vi "PCS Correlation_AVG.vi"() -> ()   [LabVIEW 2022 SP3]
uses:
  <vilib>/Analysis/baseanly.llb/Mean (DBL).vi
  <vilib>/Utility/file.llb/Write To Spreadsheet File (DBL).vi
  <vilib>/Utility/file.llb/Read From Spreadsheet File (DBL).vi
  <vilib>/Analysis/NI_AALBase.lvlib
panel:
  in  "Calc Angle":dbl=90.0
  in  "No motor":bool
  in  "No SPC":bool
  in  "stop":bool
  in  "Tab Control":T1(tab)
  out "G2 Exp Fit":cluster{dbl[], "Best Exponential Fit":dbl[]}[](graph)
  in  "AC length":i32=256
  in  "New File":bool
  in  "Total Time (s)":i32=100
  out "Time step (ms)":dbl
  in  "zero lag +":i32=1
  in  "Sample Rate (Hz)":dbl=100000.0
  in  "Data Source":enum16{"NI Card Grab", "NI File"}(ring)
  out "Cumulant ln fit":cluster{dbl[], "ln(x)/2":dbl[]}[](graph)
  out "Cumulant Fit":T2
  in  "Tau":u8
  out "bin mean":dbl format="%0.2f"
  out "Fit":T3
  out "SVM Size (um)":cluster{i32, "x":i32, dbl[][]}(graph)
  out "SVM Gaps":cluster{i32, "x":i32, dbl[][]}(graph)
  out "MultiTau":cluster{"Data out":dbl[], dbl[]}(graph)
  out "File Path":path
  out "SVM Fit Columns":T4(array[cluster])
  out "Means":dbl[](graph)
  out "Bin SD":dbl format="%0.2f"
  in  "Angle Index":u32
  out "Capture Angle":dbl
  in  "Save Path Root":path=path "D:/File"
  in  "SVs":u8
  in  "Save Bin Data":bool
  out "G2":dbl[][](graph)
  in  "Clear State":bool
  in  "angle plot":bool
  in  "Clear Chart":bool
  out "Polar Plot":picture
  out "Angle Plot":cluster{dbl[], dbl[]}(graph)
  in  "PC":T5={"Number of Bins"=1, "Bin Time (s)"=0.1, "Pause Time (s)"=1e-06}
  out "Bin Count":u32(graph)
  out "Counter":u32 caption="Counts/bin"
  out "APD saturation":bool
  in  "Run Angle collection":bool
  in  "Start":i16=90
  in  "# Steps":i16
  in  "Step Interval (degrees)":dbl=0.5 min=0.5 max=180.0 step=0.5
  out "Stop Angle":i32
  out "Current Step":i32
  out "cluster":T6
  in  "MG17Motor":refnum<k7>(container)
  in  "Diameter (um)":dbl=0.04
  out "Theory":T7
  in  "save mie":bool
  in  "Mie Input":T8={"wavlength (um)"=0.633, "Diameter (um)"=0.1, "n"=1.53, "pts"=1000.0, "Collection Angle"=4.0}
  out "Mie Theory (Matlab)":cluster{"angle":dbl[], "I":dbl[]}[](graph)
  # "SVM Method"
  # "Simple Decay Fit"
  # "Cumulant Method"
  # "Expected decay"
  # "`"
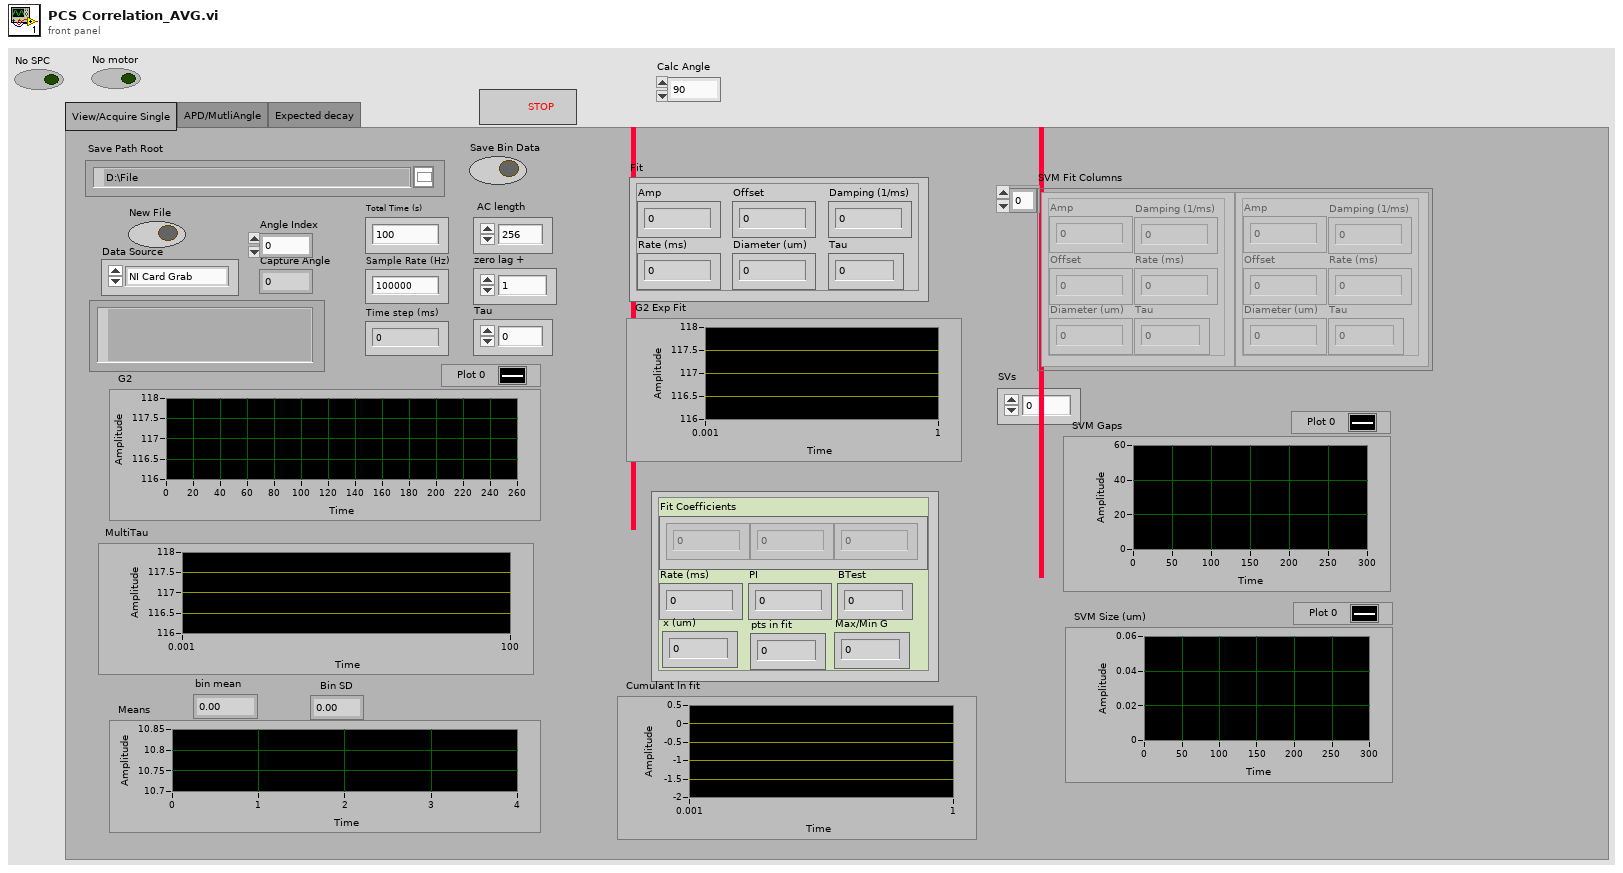
[diagram p1: front panel]
types:
  T1 = enum32{"View/Acquire Single", "APD/MutliAngle", "Expected decay"}
  T2 = cluster{"Fit Coefficients":dbl[], "Rate (ms)":dbl, "PI":dbl, "BTest":dbl, "x (um)":dbl, "pts in fit":dbl, "Max/Min G":dbl}
  T3 = cluster{"Amp":dbl, "Offset":dbl, "Damping (1/ms)":dbl, "Rate (ms)":dbl, "Diameter (um)":dbl, "Tau":dbl}
  T4 = cluster{"Amp":dbl, "Offset":dbl, "Damping (1/ms)":dbl, "Rate (ms)":dbl, "Diameter (um)":dbl, "Tau":dbl}[]
  T5 = cluster{"Number of Bins":i16, "Bin Time (s)":dbl, "Pause Time (s)":dbl}
  T6 = cluster{"running":bool, "gate active":bool, "waiting for trig":bool, "overflow":bool, "overload":bool, "overtemp":bool, "APD Sat b0":bool, "APD Sat bit1":bool, "N/A":bool, "N/A":bool, "overlow accum":bool, "overload accum":bool, "overtemp accum":bool, "APD Sat Accum 0":bool, "APD Sat Accum 0":bool}
  T7 = cluster{"Damping (1/ms)":dbl, "Rate (ms)":dbl, "Tau":dbl}
  T8 = cluster{"wavlength (um)":dbl, "Diameter (um)":dbl, "n":dbl, "pts":dbl, "Collection Angle":dbl}
  T9 = cluster{"G2 Array":dbl[][], "Sample Rate":dbl, "means":dbl[], "AC length":i32, "Total Time (s)":i32, "Angle":dbl}
  T10 = cluster{"maximum":dbl, "minimum":dbl, "clip to min":bool, "log?(F)":bool, "grid color":u32, "plot color":u32, "fmt and prec":cluster{"format":enum8{"Decimal", "Scientific", "Engineering", "Binary", "Octal", "Hex"}, "precision":u8}, "visible section":u16}
  T11 = cluster{"Boolean array[0]":bool, "Boolean array[1]":bool, "Boolean array[2]":bool, "Boolean array[3]":bool, "Boolean array[4]":bool, "Boolean array[5]":bool, "Boolean array[6]":bool, "Boolean array[7]":bool, "Boolean array[8]":bool, "Boolean array[9]":bool, "Boolean array[10]":bool, "Boolean array[11]":bool, "Boolean array[12]":bool, "Boolean array[13]":bool, "Boolean array[14]":bool}
  T12 = cluster{"Amp":dbl, "Offset":dbl, "Damping (1/ms)":dbl, "Rate (ms)":dbl, "Diameter (um)":dbl, "Tau":dbl}[][]
  T13 = cluster{"G2 Array":dbl[][], "Sample Rate":dbl, "means":dbl[], "AC length":i32, "Total Time (s)":i32, "Angle":dbl}[]
  T14 = typedef "LVBoundsTypeDef.ctl" = cluster{"Width":u32, "Height":u32}
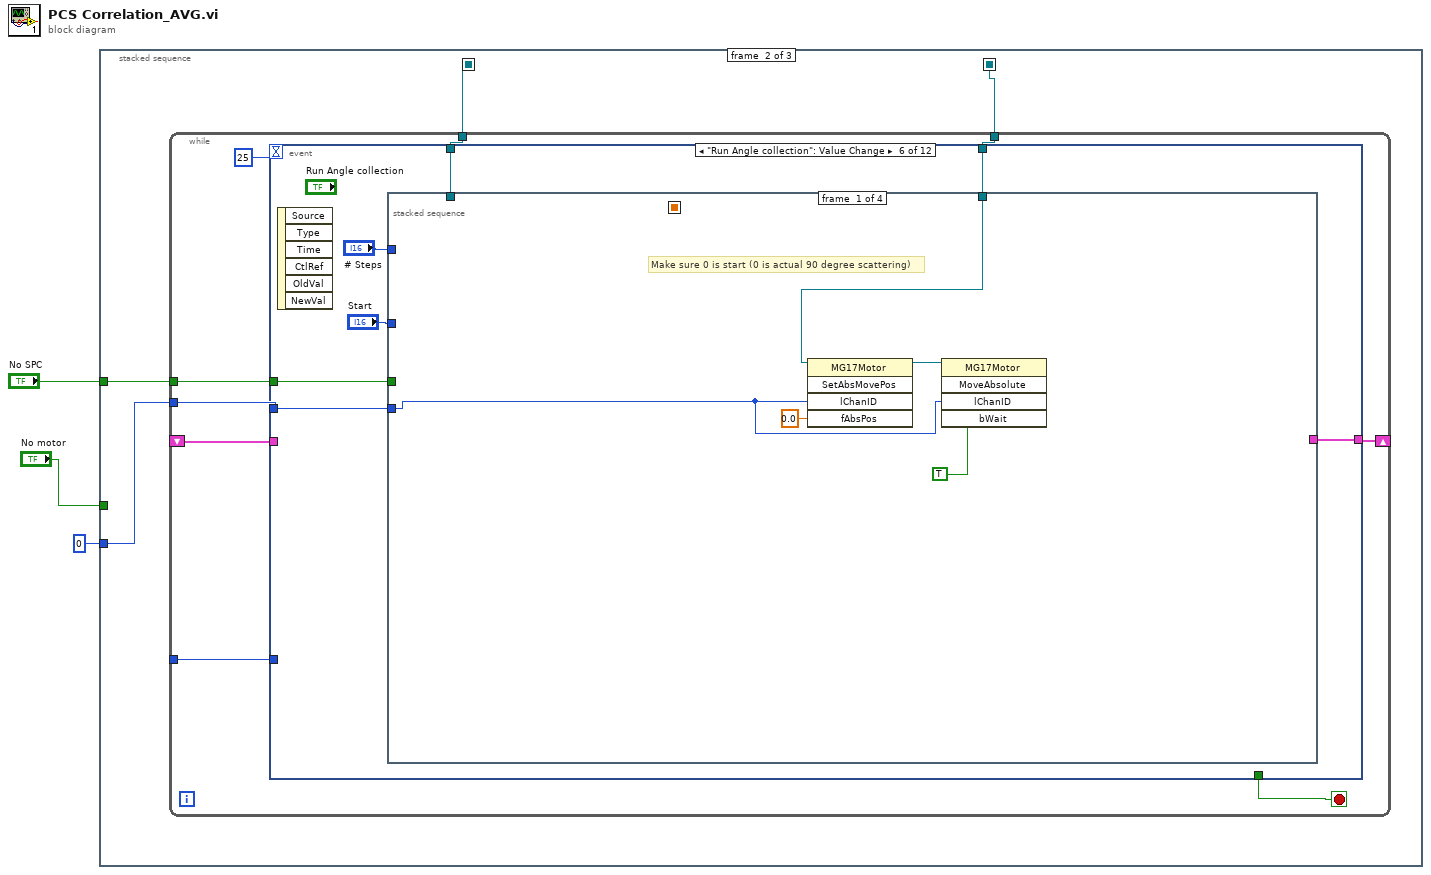
[diagram p0: block diagram]
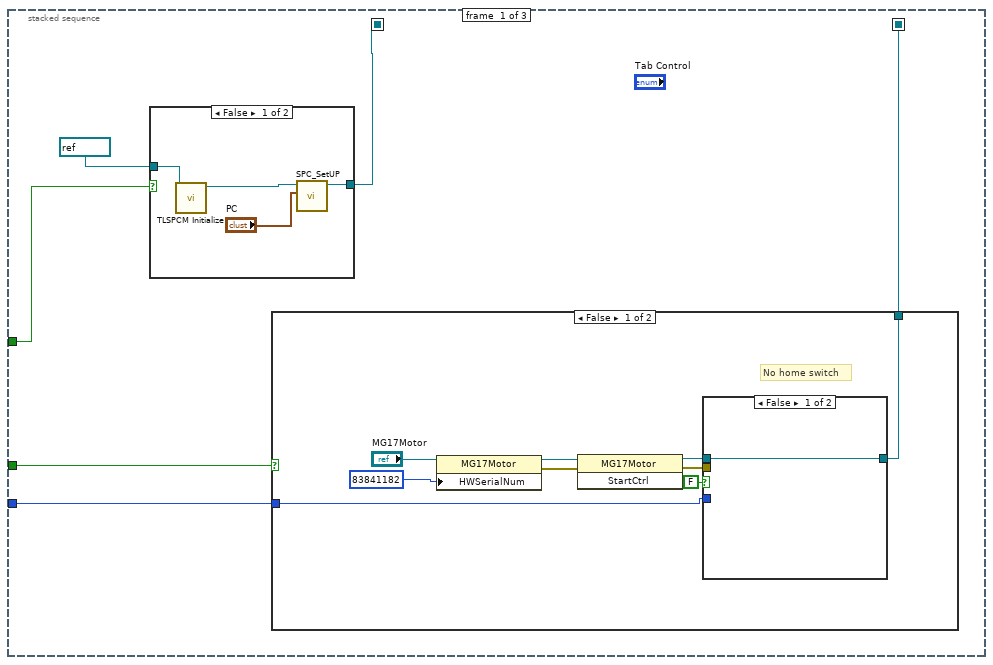
[diagram p2: hidden frame]
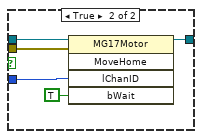
[diagram p3: hidden frame]
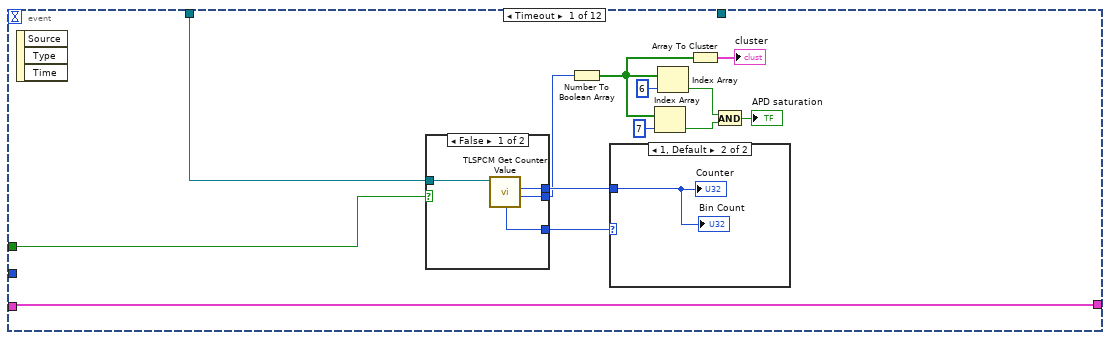
[diagram p6: hidden frame]
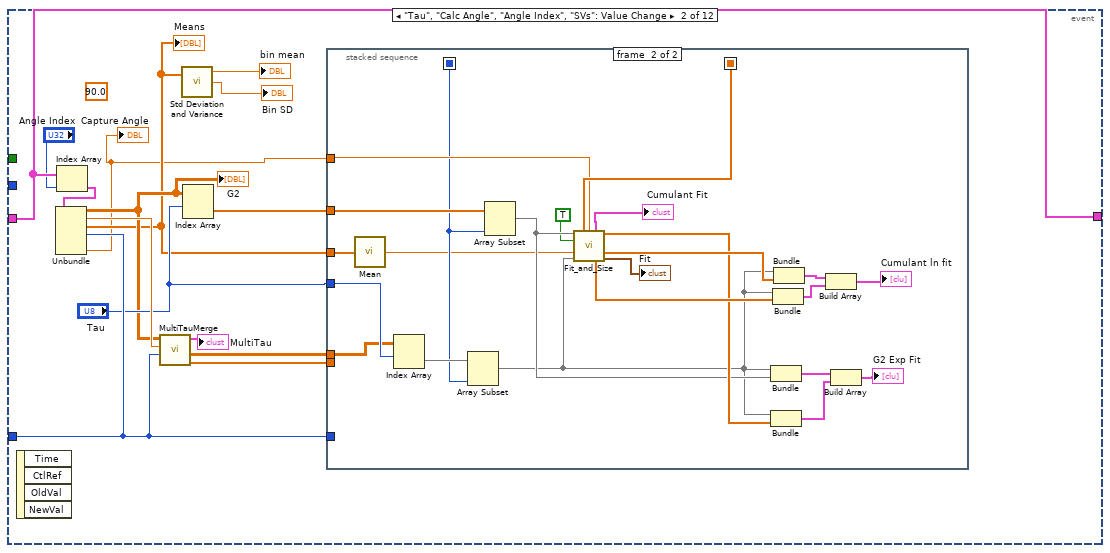
[diagram p9: hidden frame]
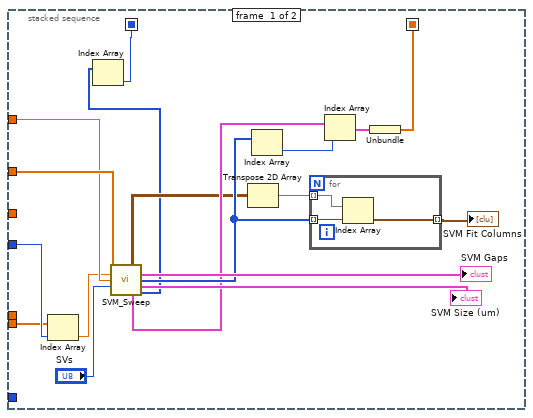
[diagram p10: hidden frame]
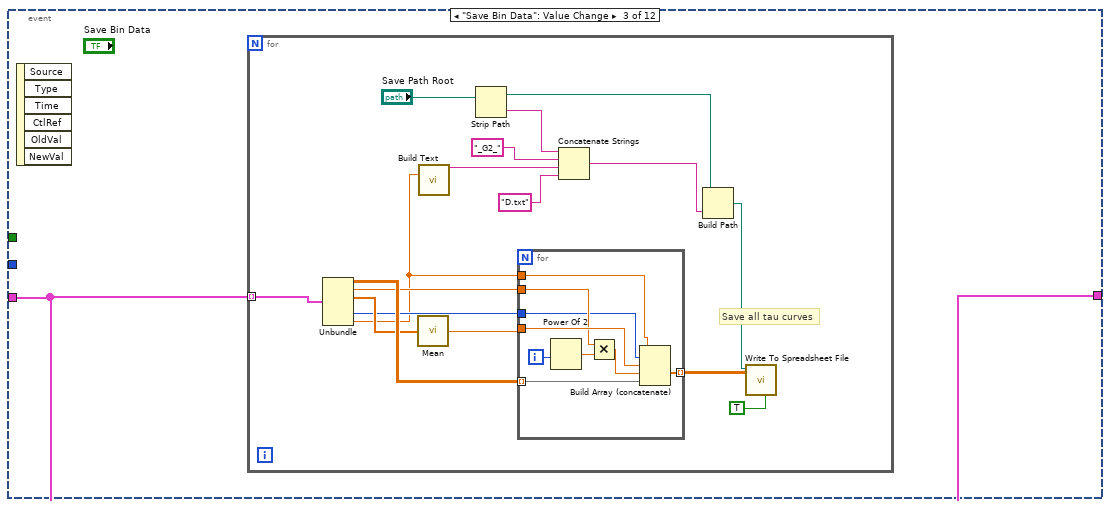
[diagram p11: hidden frame]
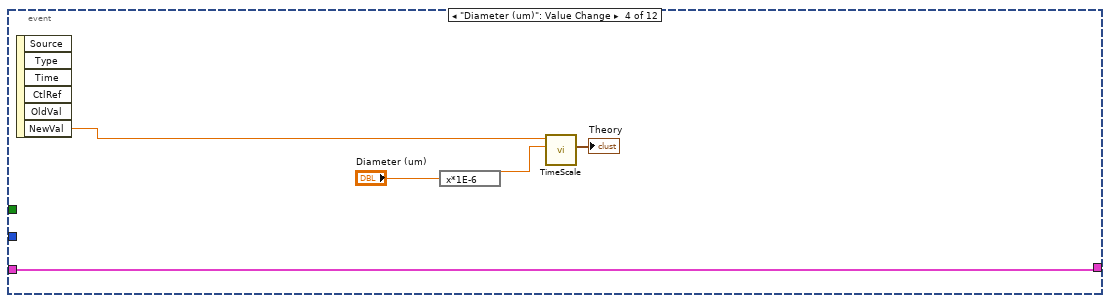
[diagram p12: hidden frame]
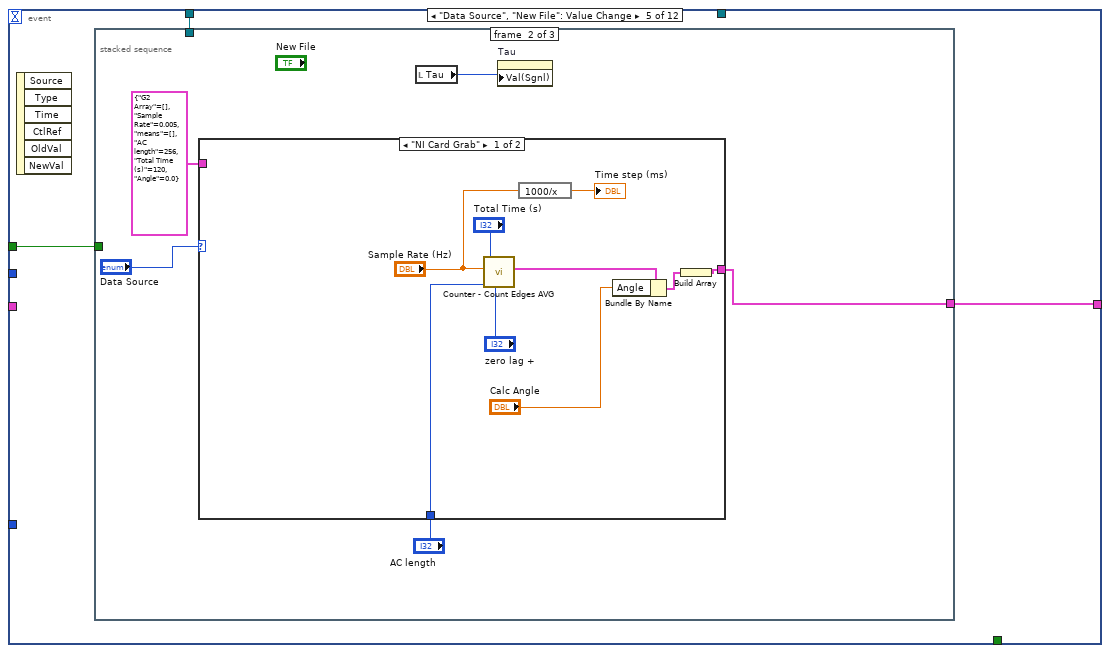
[diagram p13: hidden frame]
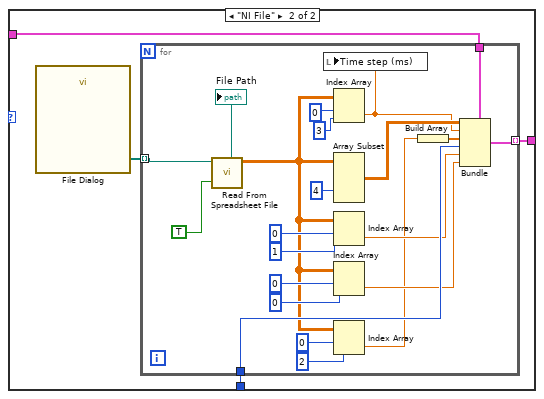
[diagram p16: hidden frame]
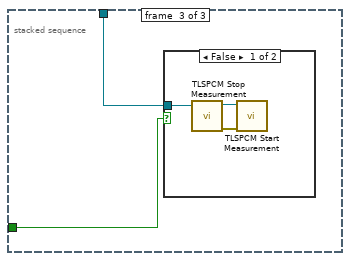
[diagram p17: hidden frame]
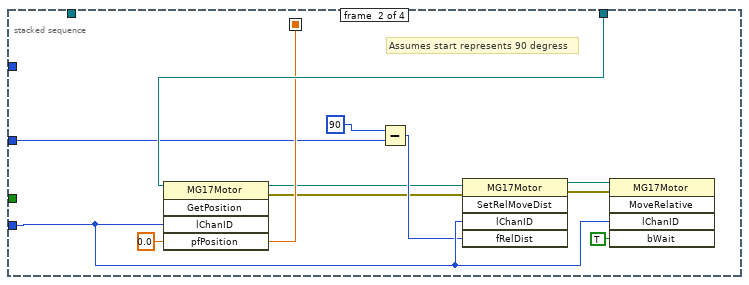
[diagram p19: hidden frame]
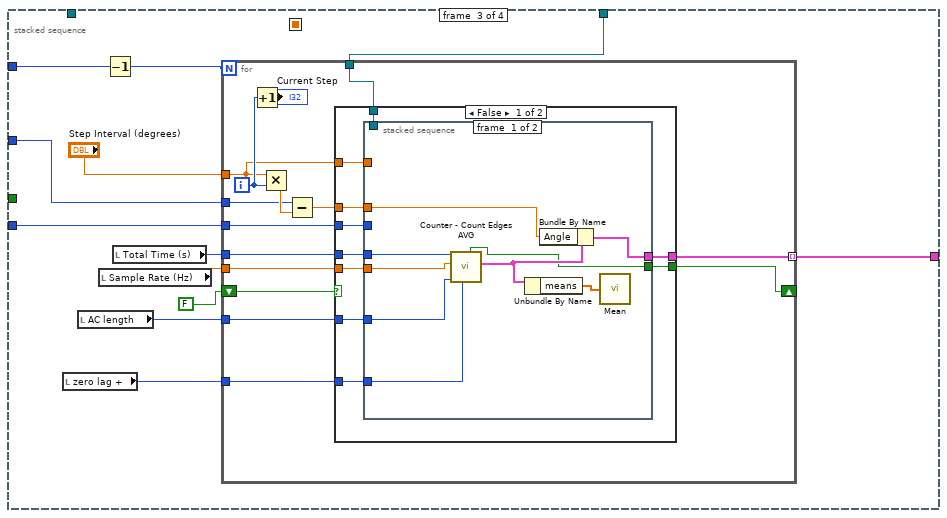
[diagram p20: hidden frame]
diagram:
  n1 = stacked-sequence {
    seq-local: [w8 _ _] -> [_ w32 w339]
    seq-local: [w7 _ _] -> [_ w31 w338]
    tunnel: 0 ("Channel A") -> [w6 w30 _]
    tunnel: "No SPC" -> [w5 w29 w337]
    tunnel: "No motor" -> [w4 _ w336]
    frame #0 {
      n2 = case shown="False" w5 {
        tunnel: refnum<visa-resource-name> "APD" ("resource name") -> [w28 _]
        tunnel: [w26 _] -> w8
        frame False {
          n3 = call <instrlib>:"TLSPCM Initialize.vi"("resource name"=w28) -> ("instrument handle out"=w27:refnum<visa-resource-name>)  [unwired: 9 in, 1 out]
          n4 = call "SPC_SetUP.vi"("PC"="PC", "VISA Refnum in"=w27) -> ("VISA Refnum out"=w26:refnum<visa-resource-name>)  [unwired: 8 in, 1 out]
        }
        frame True {
        }
      }
      n5 = case shown="False" w4 {
        tunnel: [w12 _] -> w7
        tunnel: w6 -> [w11 _]
        frame False {
          # "No home switch"
          n6 = property class="MG17Motor"(reference="MG17Motor", "HWSerialNum"=u32 83841182 ("Motor HWSerialNum A")) -> (reference out=w16:refnum<k7>, error out=w15:errorcluster)  [unwired: 1 in]
          n7 = invoke class="MG17Motor" method="StartCtrl"(reference=w16, error in=w15) -> (reference out=w14:refnum<k7>, error out=w13:errorcluster)  [unwired: 1 in, 1 out]
          n8 = case shown="False" FALSE {
            tunnel: w14 -> [w19 w24]
            tunnel: w13 -> [_ w23]
            tunnel: [w19 w21] -> w12
            tunnel: w11 -> [_ w20]
            frame False {
            }
            frame True {
              n9 = invoke class="MG17Motor" method="MoveHome"(reference=w24, error in=w23, "lChanID"=w20, "bWait"=TRUE) -> (reference out=w21:refnum<k7>)  [unwired: 1 in, 4 out]
            }
          }
        }
        frame True {
        }
      }
    }
    frame #1 {
      n10 = while {
        tunnel: [w41] -> _
        tunnel: w32 -> [w38]
        shift-right: [w36] -> _
        shift-left: _ -> [w37]
        tunnel: w31 -> [w35]
        tunnel: w30 -> [w34]
        tunnel: w29 -> [w33]
        stop <- w39 stop-if-true
        n11 = event shown="[5] \"Run Angle collection\": Value Change" {
          selector: _ -> [_ _ _ _ _ _ _ _ _ _ _ _]
          dyn-events: _ -> [_ _ _ _ _ _ _ _ _ _ _ _]
          timeout: 25 -> [_ _ _ _ _ _ _ _ _ _ _ _]
          tunnel: [_ w69 _ _ _ _ _ _ _ _ _ _] -> w41
          tunnel: [_ _ _ _ _ _ _ _ _ "stop" _ _] -> w39
          tunnel: w38 -> [w54 _ _ _ w152 w202 w291 _ w302 _ _ _]
          tunnel: w37 -> [w44 w67 w119 w147 _ _ w289 w293 w300 w303 w305 w317]
          tunnel: [w44 w67 w119 w147 w153 w207 w289 w293 w300 w303 w305 w317] -> w36
          tunnel: w35 -> [_ _ _ _ _ w206 _ _ _ _ _ _]
          tunnel: w34 -> [_ _ _ _ _ w205 _ _ _ _ _ _]
          tunnel: w33 -> [w42 _ _ _ w151 w201 w290 _ _ _ _ _]
          event Timeout {
            n12 = event-data() -> ()  [unwired: 1 in, 3 out]
            n13 = case shown="False" w42 {
              tunnel: w54 -> [w58 _]
              tunnel: [w57 _] -> w53
              tunnel: [w56 _] -> w46
              tunnel: [w55 _] -> w45
              frame False {
                n14 = call <instrlib>:"TLSPCM Get Counter Value.vi"("instrument handle"=w58) -> ("State"=w55:u16, "Counter"=w57:u32, "Index of Counter"=w56:u32)  [unwired: 6 in, 2 out]
              }
              frame True {
              }
            }
            n15 = Number To Boolean Array(number=w45) -> (Boolean array=w49:bool[])
            n16 = case shown="1, Default" w46 {
              tunnel: w53 -> [_ w59]
              frame 0 {
              }
              frame 1, Default {
                "Counter" <- w59
                "Bin Count" <- w59
              }
            }
            n17 = Index Array(array=w49, index=7) -> (element=w51:bool)
            n18 = Index Array(array=w49, index=6) -> (element=w50:bool)
            n19 = Array To Cluster(array=w49) -> (cluster=→"cluster":T11)
            n20 = And(x=w50, y=w51) -> (x .and. y?=→"APD saturation":bool)
          }
          event "Tau", "Calc Angle", "Angle Index", "SVs": Value Change {
            (unwired) 90.0 ("Angle")
            n21 = event-data() -> ()  [unwired: 1 in, 4 out]
            n22 = Index Array(array=w67, index="Angle Index") -> (element=w66:T9)
            n23 = Unbundle(w66) -> ("G2 Array"=w62:dbl[][], "Sample Rate"=w70:dbl, "means"=w61:dbl[], "AC length"=w69:i32, "Angle"=w60:dbl)  [unwired: 1 out]
            "Capture Angle" <- w60
            "G2" <- w62
            "Means" <- w61
            n24 = call "MultiTauMerge.vi"("AC length"=w69, "Time Step"=w70, "Data in"=w62) -> ("Tau Times"=w72:dbl[], "Time Array"=w71:dbl[][], "XY Graph"=→"MultiTau":cluster{dbl[], "Data out":dbl[]})  [unwired: 6 in]
            n25 = call <vilib>:"Std Deviation and Variance.vi"("X"=w61) -> ("mean"=→"bin mean":dbl, "standard deviation"=→"Bin SD":dbl)  [unwired: 1 in, 1 out]
            n26 = Index Array(array=w62, index (row)="Tau") -> (element=w74:dbl[])  [unwired: 1 in]
            n27 = stacked-sequence {
              seq-local: [w86 _] -> [_ w103]
              seq-local: [w76 _] -> [_ w97]
              tunnel: w74 -> [w90 w105]
              tunnel: w61 -> [_ w104]
              tunnel: w60 -> [w89 w102]
              tunnel: w69 -> [_ _]
              tunnel: "Tau" -> [w80 w101]
              tunnel: w72 -> [w79 _]
              tunnel: w71 -> [_ w100]
              frame #0 {
                n28 = Index Array(array=w79, index=w80) -> (element=w78:dbl)
                n29 = call "SVM_Sweep.vi"("Data IN"=w90, "time step"=w78, "Angle (degrees)"=w89, "SVs"="SVs") -> ("SVM Out Stack"=w81:T12, "SV Gaps"=→"SVM Gaps":cluster{i32, "x":i32, dbl[][]}, "Max Index"=w84:i32[], "SVM Size (um)"=→"SVM Size (um)":cluster{i32, "x":i32, dbl[][]}, "Array"=w82:cluster{"A tau":dbl[]}[], "Best Size"=w77:i32[])  [unwired: 4 in, 2 out]
                n30 = Index Array(array=w77) -> (element=w76:i32)  [unwired: 1 in]
                n31 = Transpose 2D Array(2D array=w81) -> (transposed array=w91:T12)
                n32 = Index Array(array=w84) -> (element=w85:i32)  [unwired: 1 in]
                n33 = for {
                  tunnel: w91 -> [w95] mode=indexing
                  tunnel: [w94] -> w88 mode=indexing
                  tunnel: w84 -> [w93] mode=indexing
                  n34 = Index Array(array=w95, index=w93) -> (element=w94:T3)
                }
                "SVM Fit Columns" <- w88
                n35 = Index Array(array=w82, index=w85) -> (element=w92:cluster{"A tau":dbl[]})
                n36 = Unbundle(w92) -> ("A tau"=w86:dbl[])
              }
              frame #1 {
                n37 = call-poly <vilib>:"Mean.vi"("X"=w104) -> ("mean"=w96:dbl)  [unwired: 1 out]
                n38 = Index Array(array=w100, index (row)=w101) -> (element=w99:dbl[])  [unwired: 1 in]
                n39 = Array Subset(array=w99, length=w97) -> (w98:dbl[])  [unwired: 1 in]
                n40 = Array Subset(array=w105, length=w97) -> (w107:dbl[])  [unwired: 1 in]
                n41 = call "Fit_and_Size.vi"("G2"=w107, "A tau"=w103, "Angle (degrees)"=w102, "A(tau)"=TRUE, "bin mean"=w96, "Time"=w98) -> ("Cumulant Fit"=→"Cumulant Fit":T2, "Best Exponential Fit"=w112:dbl[], "Best Polynomial Fit"=w117:dbl[], "ln(x)/2"=w116:dbl[], "Fit"=→"Fit":T3)  [unwired: 4 in, 1 out]
                n42 = Bundle(w98, w107) -> (w110:cluster{dbl[], dbl[]})  [unwired: 1 in]
                n43 = Bundle(w98, "Best Exponential Fit"=w112) -> (w111:cluster{dbl[], "Best Exponential Fit":dbl[]})  [unwired: 1 in]
                n44 = Bundle(w98, "ln(x)/2"=w116) -> (w114:cluster{dbl[], "ln(x)/2":dbl[]})  [unwired: 1 in]
                n45 = Bundle(w98, "Best Polynomial Fit"=w117) -> (w115:cluster{dbl[], "Best Polynomial Fit":dbl[]})  [unwired: 1 in]
                n46 = Build Array(w115, w114) -> (→"Cumulant ln fit":cluster{dbl[], "ln(x)/2":dbl[]}[])
                n47 = Build Array(w110, w111) -> (→"G2 Exp Fit":cluster{dbl[], "Best Exponential Fit":dbl[]}[])
              }
            }
          }
          event "Save Bin Data": Value Change {
            n48 = event-data() -> ()  [unwired: 1 in, 6 out]
            n49 = for {
              tunnel: w119 -> [w123] mode=indexing
              # "Save all tau curves"
              n50 = Unbundle(w123) -> ("G2 Array"=w134:dbl[][], "Sample Rate"=w133:dbl, "means"=w132:dbl[], "Total Time (s)"=w124:i32, "Angle"=w121:dbl)  [unwired: 1 out]
              n51 = call-poly <vilib>:"Mean.vi"("X"=w132) -> ("mean"=w122:dbl)  [unwired: 1 out]
              n52 = call "Build Text"("f"=w121) -> ("Result"=w120:string)  [unwired: 13 in, 1 out]
              n53 = Strip Path(path="Save Path Root") -> (stripped path=w126:path, name=w128:string)
              n54 = for {
                tunnel: w134 -> [w145] mode=indexing
                tunnel: [w144] -> w136 mode=indexing
                tunnel: w122 -> [w140]
                tunnel: w133 -> [w139]
                tunnel: w124 -> [w138]
                tunnel: w121 -> [w137]
                i -> [w143]
                n55 = Power Of 2(x=w143) -> (2^x=w142:dbl)
                n56 = Multiply(x=w139, y=w142) -> (x*y=w141:dbl)
                n57 = Build Array (concatenate)(w137, w138, w140, w141, w145) -> (w144:dbl[])
              }
              n58 = Concatenate Strings(w128, "_G2_" ("string"), w120, "D.txt" ("string")) -> (w127:string)
              n59 = Build Path(base path=w126, name or relative path=w127) -> (appended path=w125:path)
              n60 = call-poly <vilib>:"Write To Spreadsheet File.vi"("transpose? (no:F)"=TRUE, "2D data"=w136, "file path (dialog if empty)"=w125) -> ()  [unwired: 5 in, 1 out]
            }
          }
          event "Diameter (um)": Value Change {
            n61 = event-data() -> ("NewVal"=w146:dbl)  [unwired: 1 in, 5 out]
            n62 = expression code="x*1E-6"("Diameter (um)") -> (w149:dbl)
            n63 = call "TimeScale.vi"("Diameter (m)"=w149, "Angle (degrees)"=w146) -> ("Theory"=→"Theory":T7)  [unwired: 9 in]
          }
          event "Data Source", "New File": Value Change {
            n64 = event-data() -> ()  [unwired: 1 in, 6 out]
            n65 = stacked-sequence {
              tunnel: [_ w156 _] -> w153
              tunnel: w152 -> [w155 _ w197]
              tunnel: w151 -> [w154 _ w196]
              frame #0 {
                n66 = case shown="False" w154 {
                  tunnel: w155 -> [_ _]
                  frame False {
                  }
                  frame True {
                  }
                }
              }
              frame #1 {
                n67 = case shown="\"NI Card Grab\"" "Data Source" {
                  tunnel: "AC length" -> [w167 w173]
                  tunnel: [w164 w172] -> w156
                  tunnel: T9 {"G2 Array"=[], "Sample Rate"=0.005, "means"=[], "AC length"=256, "Total Time (s)"=120, "Angle"=0.0} ("output params") -> [_ w171]
                  frame "NI Card Grab" {
                    n68 = call "Counter - Count Edges AVG.vi"("zero lag +"="zero lag +", "AC length"=w167, "Sample Rate"="Sample Rate (Hz)", "Total Time (s)"="Total Time (s)") -> ("output params"=w163:T9)  [unwired: 4 in, 3 out]
                    n69 = expression code="1000/x"("Sample Rate (Hz)") -> (→"Time step (ms)":dbl)
                    n70 = Bundle By Name(cluster=w163, "Angle"="Calc Angle") -> (w162:T9)
                    n71 = Build Array(w162) -> (w164:T13)
                  }
                  frame "NI File" {
                    n72 = call "File Dialog"() -> ("selected paths"=w170:path[])  [unwired: 12 in, 3 out]
                    n73 = for {
                      tunnel: w173 -> [w187]
                      tunnel: w171 -> [w184]
                      tunnel: [w186] -> w172 mode=indexing
                      tunnel: w170 -> [w174] mode=indexing
                      n74 = call-poly <vilib>:"Read From Spreadsheet File.vi"("transpose (no:F)"=TRUE, "file path (dialog if empty)"=w174) -> ("all rows"=w176:dbl[][], "new file path (Not A Path if cancelled)"=→"File Path":path)  [unwired: 5 in, 3 out]
                      n75 = Index Array(array=w176, index (row)=0, index (col)=3 ("index (row)")) -> (element=w188:dbl)
                      n76 = local write "Time step (ms)"(w188) -> ()
                      n77 = Array Subset(array=w176, index (col)=4 ("index")) -> (w189:dbl[][])  [unwired: 3 in]
                      n78 = Index Array(array=w176, index (row)=0, index (col)=1 ("index (row)")) -> (element=w179:dbl)
                      n79 = Index Array(array=w176, index (row)=0, index (col)=0 ("index (row)")) -> (element=w180:dbl)
                      n80 = Index Array(array=w176, index (row)=0, index (col)=2 ("index (row)")) -> (element=w175:dbl)
                      n81 = Build Array(w175) -> (w185:dbl[])
                      n82 = Bundle(cluster=w184, "G2 Array"=w189, "Sample Rate"=w188, "means"=w185, "AC length"=w187, "Total Time (s)"=w179, "Angle"=w180) -> (w186:T9)
                    }
                  }
                }
                n83 = local read "Tau"() -> (w158:u8)
                n84 = property on="Tau" class="DigNum (strict)"("Val(Sgnl)"=w158) -> ()  [unwired: 2 in, 2 out]
              }
              frame #2 {
                n85 = case shown="False" w196 {
                  tunnel: w197 -> [w198 _]
                  frame False {
                    n86 = call <instrlib>:"TLSPCM Stop Measurement.vi"("instrument handle"=w198) -> ("error out"=w200:errorcluster, "instrument handle out"=w199:refnum<visa-resource-name>)  [unwired: 9 in]
                    n87 = call <instrlib>:"TLSPCM Start Measurement.vi"("error in (no error)"=w200, "instrument handle"=w199) -> ()  [unwired: 8 in, 2 out]
                  }
                  frame True {
                  }
                }
              }
            }
          }
          event "Run Angle collection": Value Change {
            n88 = event-data() -> ()  [unwired: 1 in, 6 out]
            n89 = stacked-sequence {
              seq-local: [_ w220 _ _] -> [_ _ _ w284]
              tunnel: [_ _ w232 _] -> w207
              tunnel: w206 -> [w208 w224 w230 w285]
              tunnel: w205 -> [w210 w219 w229 w282]
              tunnel: "Start" -> [_ w213 w228 _]
              tunnel: "# Steps" -> [_ _ w227 _]
              tunnel: w202 -> [_ _ _ w279]
              tunnel: w201 -> [_ _ _ w278]
              frame #0 {
                # "Make sure 0 is start (0 is actual 90 degree scattering)"
                n90 = invoke class="MG17Motor" method="SetAbsMovePos"(reference=w208, "lChanID"=w210, "fAbsPos"=sgl 0.0) -> (reference out=w212:refnum<k7>)  [unwired: 2 in, 4 out]
                n91 = invoke class="MG17Motor" method="MoveAbsolute"(reference=w212, "lChanID"=w210, "bWait"=TRUE) -> ()  [unwired: 2 in, 5 out]
              }
              frame #1 {
                # "Assumes start represents 90 degress"
                n92 = invoke class="MG17Motor" method="GetPosition"(reference=w224, "lChanID"=w219, "pfPosition"=sgl 0.0) -> (reference out=w217:refnum<k7>, error out=w216:errorcluster, "pfPosition"=w220:sgl)  [unwired: 2 in, 2 out]
                n93 = Subtract(x=90, y=w213) -> (x-y=w218:i32)
                n94 = invoke class="MG17Motor" method="SetRelMoveDist"(reference=w217, error in=w216, "lChanID"=w219, "fRelDist"=w218) -> (reference out=w221:refnum<k7>, error out=w215:errorcluster)  [unwired: 1 in, 3 out]
                n95 = invoke class="MG17Motor" method="MoveRelative"(reference=w221, error in=w215, "lChanID"=w219, "bWait"=TRUE) -> ()  [unwired: 1 in, 5 out]
              }
              frame #2 {
                n96 = local read "zero lag +"() -> (w233:i32)
                n97 = local read "AC length"() -> (w234:i32)
                n98 = local read "Sample Rate (Hz)"() -> (w235:dbl)
                n99 = Decrement(x=w227) -> (x-1=w225:i16)
                n100 = local read "Total Time (s)"() -> (w236:i32)
                n101 = for {
                  N: w225 -> [_]
                  tunnel: w236 -> [w251]
                  tunnel: w235 -> [w250]
                  tunnel: w234 -> [w249]
                  tunnel: w233 -> [w248]
                  tunnel: [w247] -> w232 mode=indexing
                  tunnel: "Step Interval (degrees)" -> [w241]
                  tunnel: w228 -> [w239]
                  tunnel: w230 -> [w243]
                  tunnel: w229 -> [w242]
                  shift-right: [w238] -> _
                  shift-left: FALSE -> [w237]
                  i -> [w246]
                  n102 = Increment(x=w246) -> (x+1=→"Current Step":i32)
                  n103 = Multiply(x=w241, y=w246) -> (x*y=w245:dbl)
                  n104 = Subtract(x=w239, y=w245) -> (x-y=w240:dbl)
                  n105 = case shown="False" w237 {
                    tunnel: w251 -> [w261 _]
                    tunnel: w250 -> [w260 _]
                    tunnel: w249 -> [w259 _]
                    tunnel: w248 -> [w258 _]
                    tunnel: [w257 _] -> w247
                    tunnel: w243 -> [w256 _]
                    tunnel: w242 -> [w255 _]
                    tunnel: w241 -> [w254 _]
                    tunnel: w240 -> [w253 _]
                    tunnel: [w252 TRUE ("Cancel Button out")] -> w238
                    frame False {
                      n106 = stacked-sequence {
                        tunnel: w261 -> [w270 _]
                        tunnel: w260 -> [w269 _]
                        tunnel: w259 -> [w268 _]
                        tunnel: w258 -> [w267 _]
                        tunnel: [w262 _] -> w257
                        tunnel: w254 -> [_ w273]
                        tunnel: w256 -> [_ w275]
                        tunnel: w255 -> [_ w271]
                        tunnel: w253 -> [w264 _]
                        tunnel: [w263 _] -> w252
                        frame #0 {
                          n107 = call "Counter - Count Edges AVG.vi"("zero lag +"=w267, "AC length"=w268, "Sample Rate"=w269, "Total Time (s)"=w270) -> ("output params"=w266:T9, "Cancel Button out"=w263:bool)  [unwired: 4 in, 2 out]
                          n108 = Unbundle By Name(w266) -> ("means"=w265:dbl[])
                          n109 = Bundle By Name(cluster=w266, "Angle"=w264) -> (w262:T9)
                          n110 = call-poly <vilib>:"Mean.vi"("X"=w265) -> ()  [unwired: 2 out]
                        }
                        frame #1 {
                          n111 = invoke class="MG17Motor" method="SetRelMoveDist"(reference=w275, "lChanID"=w271, "fRelDist"=w273) -> (reference out=w274:refnum<k7>)  [unwired: 2 in, 4 out]
                          n112 = invoke class="MG17Motor" method="MoveRelative"(reference=w274, "lChanID"=w271, "bWait"=TRUE) -> ()  [unwired: 2 in, 5 out]
                        }
                      }
                    }
                    frame True {
                    }
                  }
                }
              }
              frame #3 {
                n113 = case shown="False" w278 {
                  tunnel: w279 -> [w286 _]
                  frame False {
                    n114 = call <instrlib>:"TLSPCM Stop Measurement.vi"("instrument handle"=w286) -> ("error out"=w288:errorcluster, "instrument handle out"=w287:refnum<visa-resource-name>)  [unwired: 9 in]
                    n115 = call <instrlib>:"TLSPCM Start Measurement.vi"("error in (no error)"=w288, "instrument handle"=w287) -> ()  [unwired: 8 in, 2 out]
                  }
                  frame True {
                  }
                }
                n116 = local read "PC"() -> (w277:T5)
                n117 = property on="PC" class="Clust (strict)"("Val(Sgnl)"=w277) -> ()  [unwired: 2 in, 2 out]
                n118 = property on="angle plot" class="Bool (strict)"("Val(Sgnl)"="angle plot") -> ()  [unwired: 2 in, 2 out]
                n119 = invoke class="MG17Motor" method="SetAbsMovePos"(reference=w285, "lChanID"=w282, "fAbsPos"=w284) -> (reference out=w283:refnum<k7>)  [unwired: 2 in, 4 out]
                n120 = invoke class="MG17Motor" method="MoveAbsolute"(reference=w283, "lChanID"=w282, "bWait"=TRUE) -> ()  [unwired: 2 in, 5 out]
              }
            }
          }
          event "Clear State": Value Change {
            n121 = event-data() -> ()  [unwired: 1 in, 6 out]
            n122 = case shown="False" w290 {
              tunnel: w291 -> [w292 _]
              frame False {
                n123 = call <instrlib>:"TLSPCM Clear Measurement State.vi"("instrument handle"=w292) -> ()  [unwired: 9 in, 2 out]
              }
              frame True {
              }
            }
          }
          event "Step Interval (degrees)", "Start", "# Steps": Value Change {
            n124 = event-data() -> ()  [unwired: 1 in, 6 out]
            n125 = local read "Step Interval (degrees)"() -> (w298:dbl)
            n126 = local read "# Steps"() -> (w299:i16)
            n127 = local read "Start"() -> (w297:i16)
            n128 = Decrement(x=w299) -> (x-1=w294:i16)
            n129 = Multiply(x=w298, y=w294) -> (x*y=w296:dbl)
            n130 = Subtract(x=w297, y=w296) -> (x-y=→"Stop Angle":dbl)
          }
          event "PC": Value Change {
            n131 = event-data() -> ("NewVal"=w301:T5)  [unwired: 1 in, 5 out]
            n132 = call "SPC_SetUP.vi"("PC"=w301, "VISA Refnum in"=w302) -> ()  [unwired: 8 in, 2 out]
          }
          event "stop": Value Change {
            n133 = event-data() -> ()  [unwired: 1 in, 6 out]
          }
          event "Clear Chart": Value Change {
            n134 = event-data() -> ()  [unwired: 1 in, 6 out]
            n135 = property on="Bin Count" class="WFChart (strict)"("History Data"=u32[] []) -> ()  [unwired: 2 in, 2 out]
          }
          event "angle plot", "save mie", "Mie Input": Value Change {
            n136 = event-data() -> ()  [unwired: 1 in, 6 out]
            n137 = for {
              tunnel: w317 -> [w335] mode=indexing
              tunnel: [w333] -> w309 mode=indexing
              tunnel: [w332] -> w312 mode=indexing
              tunnel: [w331] -> w318 mode=indexing
              n138 = Unbundle By Name(w335) -> ("Angle"=w333:dbl, "means"=w334:dbl[])
              n139 = call-poly <vilib>:"Mean.vi"("X"=w334) -> ("mean"=w332:dbl)  [unwired: 1 out]
              n140 = Bundle("mean"=w332, "Angle"=w333) -> (w331:cluster{"mean":dbl, "Angle":dbl})  [unwired: 1 in]
            }
            n141 = local write "angle plot"(FALSE ("angle plot")) -> ()
            n142 = property on="Polar Plot" class="Pict"() -> ("Draw Area Size"=w322:T14)  [unwired: 2 in, 2 out]
            n143 = Bundle(w309, w312) -> (→"Angle Plot":cluster{dbl[], dbl[]})  [unwired: 1 in]
            n144 = call <vilib>:"Polar Plot with Point Options.vi"("data array [mag, phase (deg)]"=w318, "dimensions (w,h)"=w322, "polar attributes"=T10 {"maximum"=0.0, "minimum"=0.0, "clip to min"=FALSE, "log?(F)"=FALSE, "grid color"=6710886, "plot color"=16711680, "fmt and prec"={"format"=enum."Decimal", "precision"=0}, "visible section"=4}, "Size"=u16 3) -> ("new picture"=→"Polar Plot":picture)  [unwired: 11 in]
            n145 = flat-sequence {
              tunnel: "Mie Input" -> [_]
              tunnel: [dbl[] [] ("angle")] -> w311
              tunnel: [dbl[][] [] ("I")] -> w310
              tunnel: w309 -> [_]
              frame #0 {
              }
            }
            n146 = for {
              tunnel: [w325] -> w307 mode=indexing
              tunnel: w311 -> [w324]
              tunnel: w310 -> [w323] mode=indexing
              n147 = Bundle("angle"=w324, "I"=w323) -> (w325:cluster{"angle":dbl[], "I":dbl[]})  [unwired: 1 in]
            }
            "Mie Theory (Matlab)" <- w307
            n148 = Build Array (concatenate)(w311, w310, w309, w312) -> (w315:dbl[][])
            n149 = case shown="True" "save mie" {
              tunnel: w315 -> [_ w330]
              frame False {
              }
              frame True {
                n150 = call-poly <vilib>:"Write To Spreadsheet File.vi"("transpose? (no:F)"=TRUE, "format (%.3f)"="%.3e", "2D data"=w330) -> ()  [unwired: 5 in, 1 out]
              }
            }
          }
        }
      }
    }
    frame #2 {
      n151 = case shown="False" w337 {
        tunnel: w339 -> [w341 _]
        frame False {
          n152 = call <instrlib>:"TLSPCM Close.vi"("instrument handle"=w341) -> ()  [unwired: 10 in, 1 out]
        }
        frame True {
        }
      }
      n153 = case shown="False" w336 {
        tunnel: w338 -> [w340 _]
        frame False {
          n154 = invoke class="MG17Motor" method="StopCtrl"(reference=w340) -> ()  [unwired: 2 in, 3 out]
        }
        frame True {
        }
      }
    }
  }
